vi "Experiment with Grid Generation.vi"(6 "Pixel Boundary (in pixels)":cluster{"Tot Y Pixels":i32, "Tot X Pixels":i32}, 7 "Field Of View (in metres)":T2={"X FOV (in metres)"=0.0007, "Y FOV (in metres)"=0.0007}, 9 "Pixel Offsets":T3, 10 "Grid Spacing (in metres)":T1, 11 "Grid Dimensions":cluster{"X-Dimension":i32, "Y-Dimension":i32}) -> (0 "Array of Y coordinates":i32[](array[numeric]), 1 "Array of X coordinates":i32[](array[numeric]), 3 "Grid OUT (in X-Y pixels)":cluster{"Y":i32, "X":i32}[](array[cluster]))   [LabVIEW 2012]
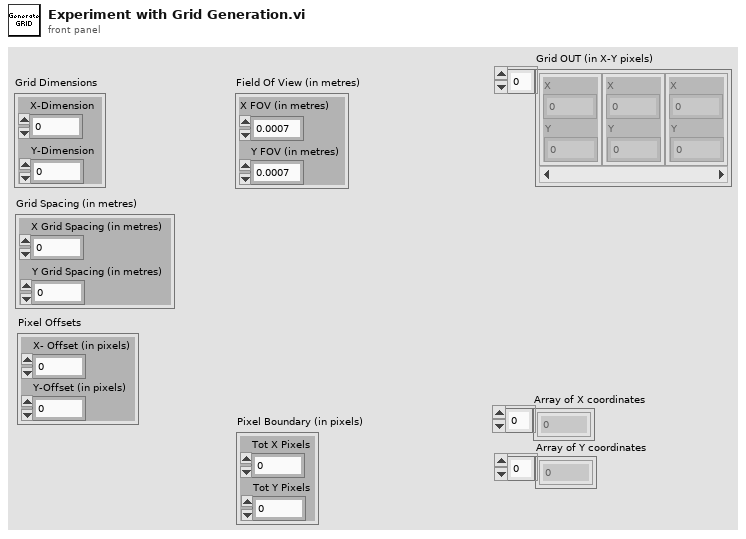
[diagram p1: front panel]
types:
  T1 = cluster{"X Grid Spacing (in metres)":dbl, "Y Grid Spacing (in metres)":dbl}
  T2 = cluster{"X FOV (in metres)":dbl, "Y FOV (in metres)":dbl}
  T3 = cluster{"X- Offset (in pixels)":i32, "Y-Offset (in pixels)":i32}
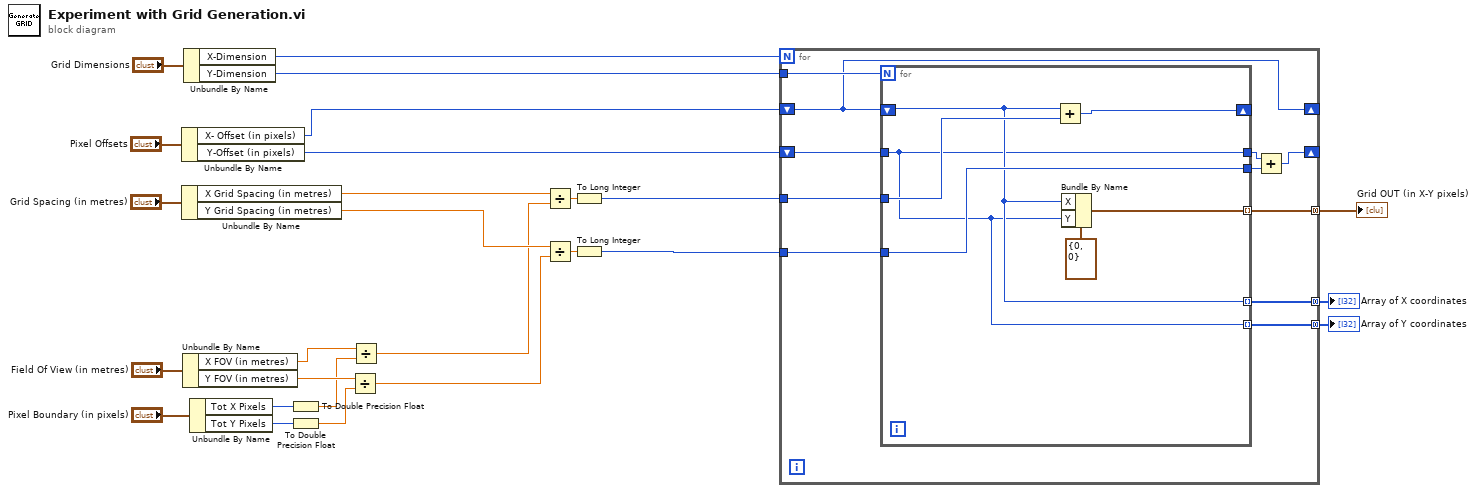
[diagram p0: block diagram]
diagram:
  n1 = Unbundle By Name("Pixel Offsets") -> ("X- Offset (in pixels)"=w3:i32, "Y-Offset (in pixels)"=w4:i32)
  n2 = Unbundle By Name("Grid Spacing (in metres)") -> ("X Grid Spacing (in metres)"=w13:dbl, "Y Grid Spacing (in metres)"=w12:dbl)
  n3 = Unbundle By Name("Field Of View (in metres)") -> ("X FOV (in metres)"=w24:dbl, "Y FOV (in metres)"=w23:dbl)
  n4 = Unbundle By Name("Grid Dimensions") -> ("X-Dimension"=w17:i32, "Y-Dimension"=w16:i32)
  n5 = Unbundle By Name("Pixel Boundary (in pixels)") -> ("Tot X Pixels"=w22:i32, "Tot Y Pixels"=w21:i32)
  n6 = To Double Precision Float(number=w22) -> (double precision float=w20:dbl)
  n7 = To Double Precision Float(number=w21) -> (double precision float=w19:dbl)
  n8 = Divide(x=w23, y=w19) -> (x/y=w11:dbl)
  n9 = Divide(x=w24, y=w20) -> (x/y=w10:dbl)
  n10 = Divide(x=w13, y=w10) -> (x/y=w9:dbl)
  n11 = Divide(x=w12, y=w11) -> (x/y=w8:dbl)
  n12 = To Long Integer(number=w9) -> (32bit integer=w7:i32)
  n13 = To Long Integer(number=w8) -> (32bit integer=w6:i32)
  n14 = for {
    N: w17 -> [_]
    tunnel: w16 -> [w37]
    tunnel: w7 -> [w36]
    tunnel: w6 -> [w35]
    shift-right: [w27] -> _
    shift-left: w3 -> [w27]
    shift-right: [w30] -> _
    shift-left: w4 -> [w34]
    tunnel: [w33] -> w5 mode=concatenating
    tunnel: [w29] -> w2 mode=concatenating
    tunnel: [w28] -> w1 mode=concatenating
    n15 = for {
      N: w37 -> [_]
      tunnel: w36 -> [w40]
      tunnel: w35 -> [w41]
      tunnel: w34 -> [w38]
      tunnel: [w43] -> w33 mode=indexing
      shift-right: [w42] -> _
      shift-left: w27 -> [w39]
      tunnel: [w38] -> w32
      tunnel: [w41] -> w31
      tunnel: [w39] -> w29 mode=indexing
      tunnel: [w38] -> w28 mode=indexing
      n16 = Add(x=w39, y=w40) -> (x+y=w42:i32)
      n17 = Bundle By Name(cluster=cluster{"X":i32, "Y":i32} {"X"=0, "Y"=0} ("Grid OUT"), "X"=w39, "Y"=w38) -> (w43:cluster{"X":i32, "Y":i32})
    }
    n18 = Add(x=w32, y=w31) -> (x+y=w30:i32)
  }
  "Grid OUT (in X-Y pixels)" <- w5
  "Array of X coordinates" <- w2
  "Array of Y coordinates" <- w1
